vi "FixPegInWay.vi"(11 "Sorted Data":dbl[][](array[numeric])) -> (3 "Sorted Data 2":dbl[][](array[numeric]))   [LabVIEW 2016]
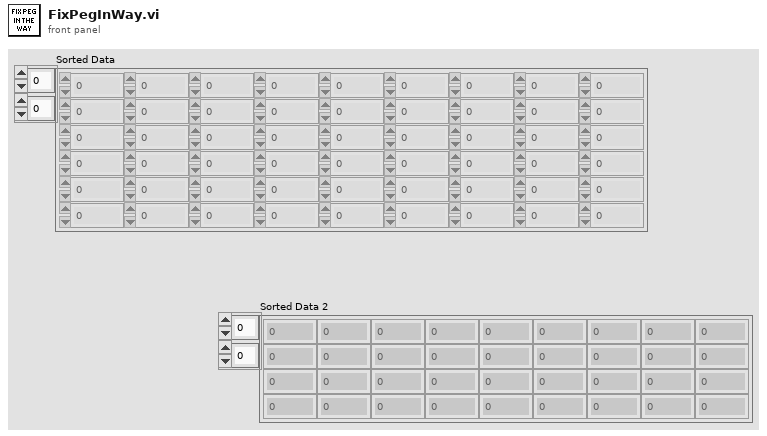
[diagram p1: front panel]
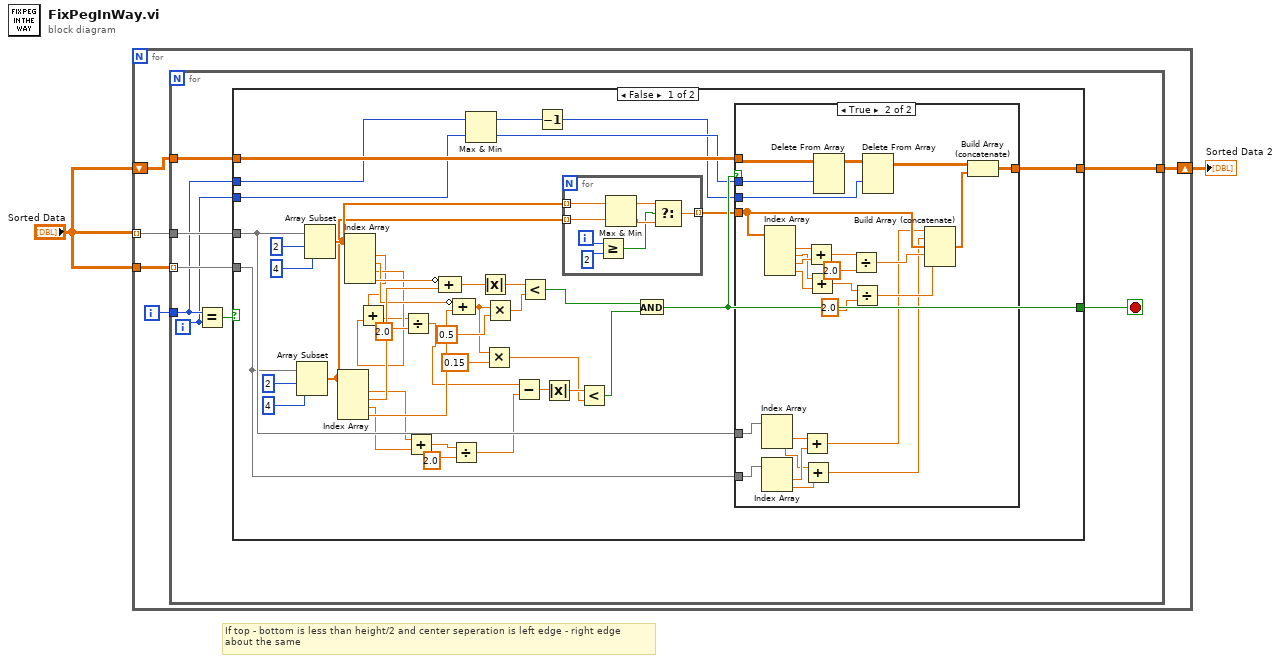
[diagram p0: block diagram]
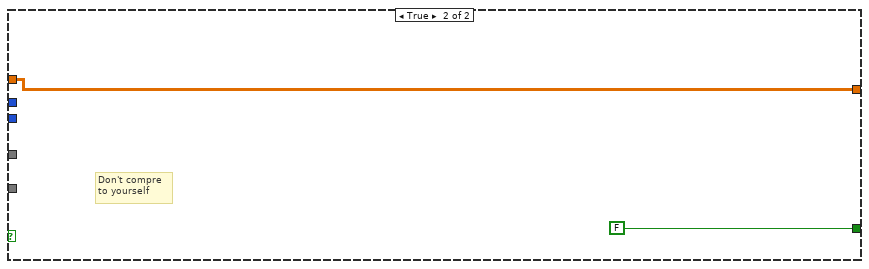
[diagram p3: hidden frame]
diagram:
  # "If top - bottom is less than height/2 and center seperation is left edge - right edge\nabout the same"
  n1 = for {
    tunnel: "Sorted Data" -> [w7] mode=indexing
    tunnel: "Sorted Data" -> [w6]
    shift-right: [w3] -> w1
    shift-left: "Sorted Data" -> [w4]
    i -> [w5]
    n2 = for {
      tunnel: w7 -> [w15]
      tunnel: w6 -> [w13] mode=indexing
      tunnel: w5 -> [w11]
      tunnel: w4 -> [w12]
      tunnel: [w9] -> w3
      i -> [w10]
      stop <- w8 stop-if-true
      n3 = Equal?(x=w11, y=w10) -> (x = y?=w14:bool)
      n4 = case shown="False" w14 {
        tunnel: w15 -> [w28 _]
        tunnel: w13 -> [w27 _]
        tunnel: [w37 FALSE] -> w8
        tunnel: w12 -> [w38 w93]
        tunnel: w11 -> [w34 _]
        tunnel: w10 -> [w26 _]
        tunnel: [w35 w93] -> w9
        frame False {
          n5 = Array Subset(array=w27, index=2, length=4) -> (w29:dbl[])
          n6 = Array Subset(array=w28, index=2, length=4) -> (w30:dbl[])
          n7 = Index Array(array=w29) -> (element #1=w20:dbl, element #2=w52:dbl, element #3=w19:dbl, element #4=w50:dbl)  [unwired: 4 in]
          n8 = Index Array(array=w30) -> (element #1=w22:dbl, element #2=w51:dbl, element #3=w24:dbl, element #4=w53:dbl)  [unwired: 4 in]
          n9 = Add(x=w22, y=w24) -> (x+y=w23:dbl)
          n10 = Divide(x=w23, y=2.0) -> (x/y=w21:dbl)
          n11 = Add(x=w20, y=w19) -> (x+y=w18:dbl)
          n12 = Compound Arithmetic op=ADD(invert w53, w52) -> (w40:dbl)
          n13 = Divide(x=w18, y=2.0) -> (x/y=w16:dbl)
          n14 = Compound Arithmetic op=ADD(invert w51, w50) -> (w44:dbl)
          n15 = Max & Min(x=w34, y=w26) -> (max(x,y)=w32:i32, min(x,y)=w33:i32)
          n16 = Absolute Value(x=w40) -> (abs(x)=w39:dbl)
          n17 = Multiply(x=w44, y=0.15) -> (x*y=w42:dbl)
          n18 = Multiply(x=w44, y=0.5) -> (x*y=w49:dbl)
          n19 = Subtract(x=w21, y=w16) -> (x-y=w46:dbl)
          n20 = Less?(x=w39, y=w49) -> (x < y?=w48:bool)
          n21 = Decrement(x=w32) -> (x-1=w31:i32)
          n22 = Absolute Value(x=w46) -> (abs(x)=w45:dbl)
          n23 = for {
            tunnel: w30 -> [w92] mode=indexing
            tunnel: w29 -> [w91] mode=indexing
            tunnel: [w85] -> w36 mode=indexing
            i -> [w89]
            n24 = Greater Or Equal?(x=w89, y=2) -> (x >= y?=w86:bool)
            n25 = Max & Min(x=w92, y=w91) -> (max(x,y)=w88:dbl, min(x,y)=w87:dbl)
            n26 = Select(t=w88, s=w86, f=w87) -> (s? t:f=w85:dbl)
          }
          n27 = Less?(x=w45, y=w42) -> (x < y?=w41:bool)
          n28 = And(x=w48, y=w41) -> (x .and. y?=w37:bool)
          n29 = case shown="True" w37 {
            tunnel: w38 -> [w58 w84]
            tunnel: w33 -> [_ w83]
            tunnel: w31 -> [_ w81]
            tunnel: w36 -> [_ w70]
            tunnel: [w58 w79] -> w35
            tunnel: w28 -> [_ w66]
            tunnel: w27 -> [_ w65]
            frame False {
            }
            frame True {
              n30 = Index Array(array=w66) -> (element #1=w64:dbl, element #2=w62:dbl)  [unwired: 2 in]
              n31 = Index Array(array=w65) -> (element #1=w63:dbl, element #2=w61:dbl)  [unwired: 2 in]
              n32 = Index Array(array=w70) -> (element #1=w77:dbl, element #2=w76:dbl, element #3=w78:dbl, element #4=w75:dbl)  [unwired: 4 in]
              n33 = Add(x=w64, y=w63) -> (x+y=w60:dbl)
              n34 = Add(x=w62, y=w61) -> (x+y=w59:dbl)
              n35 = Add(x=w77, y=w78) -> (x+y=w74:dbl)
              n36 = Add(x=w76, y=w75) -> (x+y=w73:dbl)
              n37 = Delete From Array(array=w84, index (row)=w83) -> (array with subset deleted=w82:dbl[][])  [unwired: 2 in, 1 out]
              n38 = Divide(x=w74, y=2.0) -> (x/y=w69:dbl)
              n39 = Divide(x=w73, y=2.0) -> (x/y=w68:dbl)
              n40 = Delete From Array(array=w82, index (row)=w81) -> (array with subset deleted=w80:dbl[][])  [unwired: 2 in, 1 out]
              n41 = Build Array (concatenate)(w60, w59, w70, w69, w68) -> (w67:dbl[])
              n42 = Build Array (concatenate)(w80, w67) -> (w79:dbl[][])
            }
          }
        }
        frame True {
          # "Don't compre\nto yourself"
        }
      }
    }
  }
  "Sorted Data 2" <- w1
